vi "RCstage_Test_Hm.vi"(2 "error in":errorcluster, 4 "Stage Ref.  In":refnum<visa-resource-name>="Lf_Tester_Stage") -> (0 "error out":errorcluster, 1 "Stage Ref. Out":refnum<visa-resource-name>="Lf_Tester_Stage")   [LabVIEW 2017]
panel:
  # "1.PIO switch on\n2.Servo on\n3.Home \n4.Move to Pos"
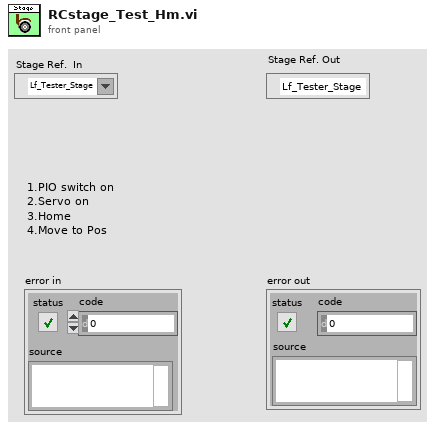
[diagram p1: front panel]
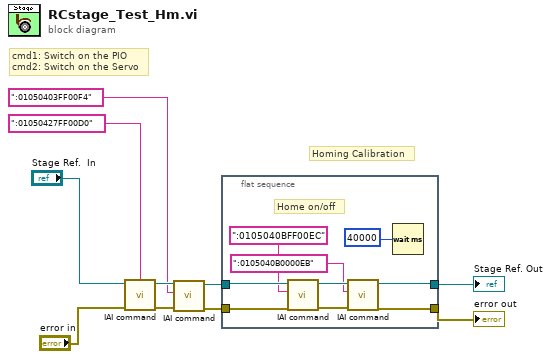
[diagram p0: block diagram]
diagram:
  # "Homing Calibration"
  # "cmd1: Switch on the PIO\ncmd2: Switch on the Servo"
  n1 = call "IAI command.vi"("error in (no error)"="error in", "packet"=":01050427FF00D0", "VISA Refnum in"="Stage Ref.  In") -> ("error out"=w7:errorcluster, "VISA Refnum"=w8:refnum<visa-resource-name>)  [unwired: 6 in, 1 out]
  n2 = call "IAI command.vi"("error in (no error)"=w7, "packet"=":01050403FF00F4", "VISA Refnum in"=w8) -> ("error out"=w4:errorcluster, "VISA Refnum"=w3:refnum<visa-resource-name>)  [unwired: 6 in, 1 out]
  n3 = flat-sequence {
    tunnel: w4 -> [w13]
    tunnel: [w16] -> w2
    tunnel: w3 -> [w14]
    tunnel: [w15] -> w1
    frame #0 {
      # "Home on/off"
      n4 = call "IAI command.vi"("error in (no error)"=w13, "packet"=":0105040BFF00EC", "VISA Refnum in"=w14) -> ("error out"=w18:errorcluster, "VISA Refnum"=w17:refnum<visa-resource-name>)  [unwired: 6 in, 1 out]
      n5 = call "IAI command.vi"("error in (no error)"=w18, "packet"=":0105040B0000EB", "VISA Refnum in"=w17) -> ("error out"=w16:errorcluster, "VISA Refnum"=w15:refnum<visa-resource-name>)  [unwired: 6 in, 1 out]
      n6 = Wait (ms)(milliseconds to wait=u32 40000) -> ()  [unwired: 1 out]
    }
  }
  "error out" <- w2
  "Stage Ref. Out" <- w1
